vi "Convert Num to Ohms.vi"(1 "String":string) -> (0 "Numeric":dbl)   [LabVIEW 2013]
panel:
  out "Numeric (SI Notation)":dbl format="%#_6p"
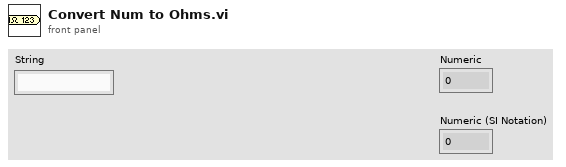
[diagram p1: front panel]
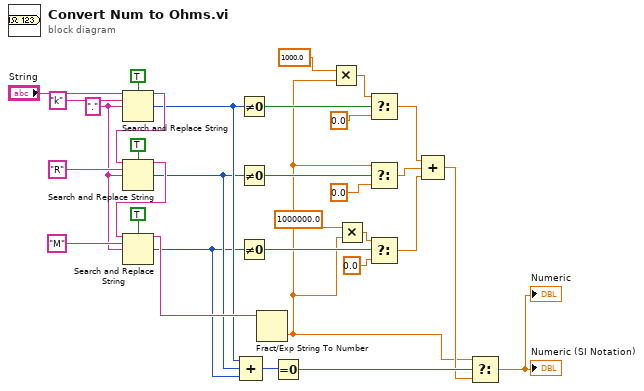
[diagram p0: block diagram]
diagram:
  w23 = "." ("replace string (\"\")")
  n1 = Search and Replace String(case sensitive?=TRUE ("ignore case? (F)"), input string="String", search string="k", replace string=w23) -> (result string=w27:string, number of replacements=w8:i32)  [unwired: 4 in, 2 out]
  n2 = Search and Replace String(case sensitive?=TRUE ("ignore case? (F)"), input string=w27, search string="R", replace string=w23) -> (result string=w24:string, number of replacements=w7:i32)  [unwired: 4 in, 2 out]
  n3 = Search and Replace String(case sensitive?=TRUE ("ignore case? (F)"), input string=w24, search string="M", replace string=w23) -> (result string=w10:string, number of replacements=w6:i32)  [unwired: 4 in, 2 out]
  n4 = Not Equal To 0?(x=w8) -> (x != 0?=w22:bool)
  n5 = Not Equal To 0?(x=w7) -> (x != 0?=w21:bool)
  n6 = Not Equal To 0?(x=w6) -> (x != 0?=w20:bool)
  n7 = Compound Arithmetic op=ADD(w8, w7, w6) -> (w5:i32)
  n8 = Fract/Exp String To Number(string=w10) -> (number=w2:dbl)  [unwired: 3 in, 1 out]
  n9 = Equal To 0?(x=w5) -> (x = 0?=w4:bool)
  n10 = Multiply(x=1000.0, y=w2) -> (x*y=w19:dbl)
  n11 = Multiply(x=1000000.0, y=w2) -> (x*y=w14:dbl)
  n12 = Select(t=w19, s=w22, f=0.0) -> (s? t:f=w11:dbl)
  n13 = Select(t=w2, s=w21, f=0.0) -> (s? t:f=w13:dbl)
  n14 = Select(t=w14, s=w20, f=0.0) -> (s? t:f=w12:dbl)
  n15 = Compound Arithmetic op=ADD(w11, w13, w12) -> (w3:dbl)
  n16 = Select(t=w2, s=w4, f=w3) -> (s? t:f=→"Numeric" →"Numeric (SI Notation)":dbl)
